vi "io_read_errors.vi"(8 "error in":errorcluster, 11 "VISA resource name":refnum<visa-resource-name>) -> (0 "error out":errorcluster, 3 "VISA resource name out":refnum<visa-resource-name>)   [LabVIEW 2014, in "rszvl_rsidr_core.lvlib"]
uses:
  rszvl_rsidr_core.lvlib
  type_Error_Codes.ctl
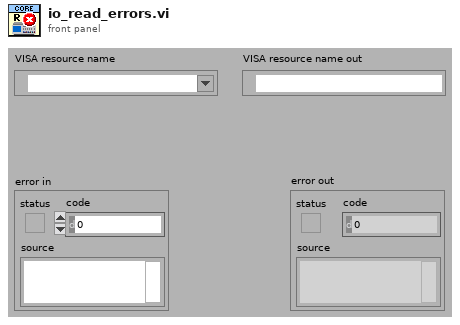
[diagram p1: front panel]
types:
  T1 = typedef "rszvl_rsidr_core.lvlib/type_Error_Codes.ctl" = enum16{"No_error", "VISA_err_ResourceNotFound", "VISA_err_Timeout", "VISA_warn_MoreDataAvailable", "RS_err_MissingCallback", "RS_err_InvalidAttribute", "RS_err_InvalidValue", "RS_err_UnknownResource", "RS_err_AlreadyInitialized", "RS_err_InstrumentStatus", "RS_err_BadRepCapName", "RS_err_TypesMismatch", "RS_err_ValueNotSupported", "RS_err_InvalidRngTable", "RS_err_IDqueryFail", "RS_err_UnexpResponse", "VISA_warn_ConfigNotLoaded", "RS_err_AttributeNotReadable", "RS_err_AttributeNotWritable", "RS_err_InstrumentType", "RS_err_InstrumentOption", "VISA_err_InvalidSize", "RS_err_ReliabilityIndicator", "VISA_warn_UnknownStatus", "VISA_warn_TermCharRead", "VISA_err_IO_error"}
  T2 = typedef "rszvl_rsidr_core.lvlib/type_Session_Data.ctl" = cluster{"Instr type":string, "Instr type for err. msg.":string, "Installed Options":string[], "OPC Timeout":i32, "Query Instrument Status":bool, "Check Range":bool, "Check Options":bool, "Add LF to Write":bool, "Simulate":bool, "Logging":bool, "Logging params":variant, "Interface Type":enum16{"Unknown", "GPIB", "VXI", "GPIB_VXI", "ASRL", "PXI", "TCPIP", "USB", "SOCKET"}, "Fast Sweep":i32, "AdditionalFlags":i32, "WaitBeforeWrite":i32, "WaitBeforeRead":i32, "BinDataChunkSize":i64}
  T3 = enum16{"Unknown", "GPIB", "VXI", "GPIB_VXI", "ASRL", "PXI", "TCPIP", "USB", "SOCKET"}
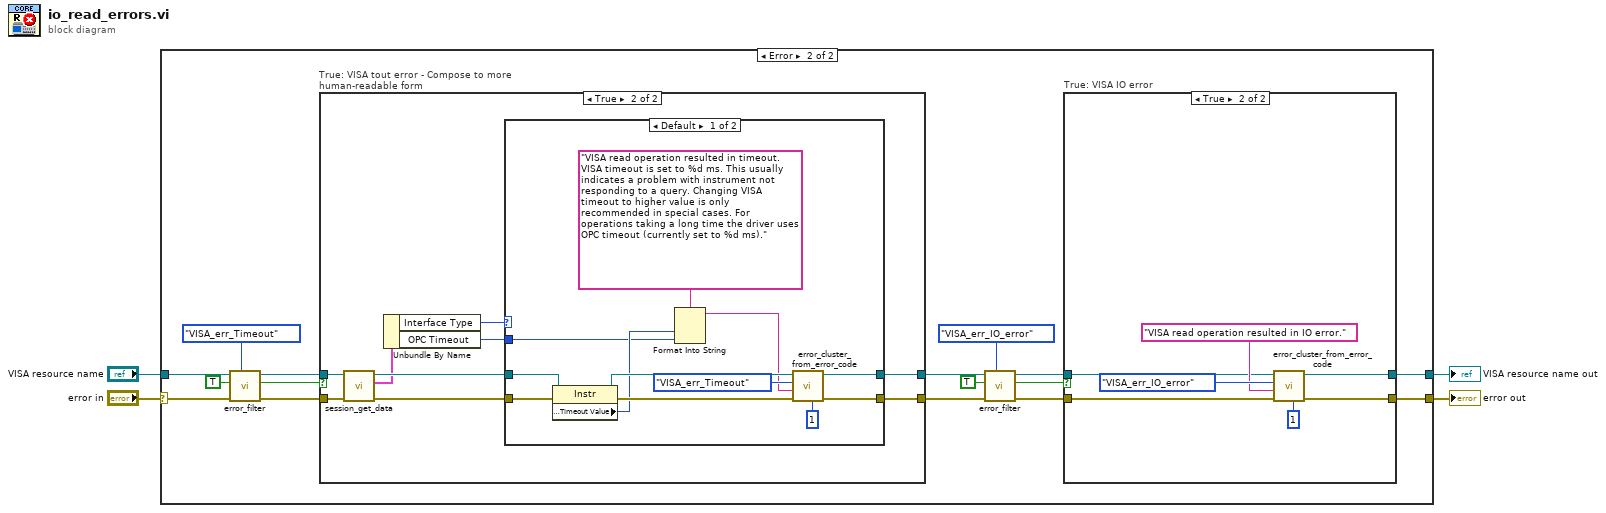
[diagram p0: block diagram]
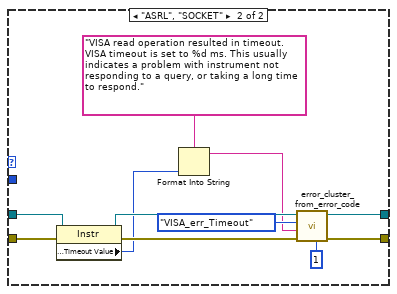
[diagram p5: hidden frame]
diagram:
  n1 = case shown="Error" "error in" {
    selector: "error in" -> [w6 w18]
    tunnel: [w6 w7] -> w2
    tunnel: "VISA resource name" -> [w5 w17]
    tunnel: [w5 w8] -> w1
    frame No Error {
    }
    frame Error {
      n2 = call "error_filter.vi"("Error Enum in"=type_Error_Codes."VISA_err_Timeout" ("Code to detect"), "error in"=w18, "Clear detected code (F)"=TRUE, "VISA resource name"=w17) -> ("error out"=w20:errorcluster, "Code Detected"=w19:bool, "VISA resource name out"=w16:refnum<visa-resource-name>)  [unwired: 5 in]
      n3 = case "True: VISA tout error - Compose to more human-readable form" shown="True" w19 {
        tunnel: w20 -> [w33 w40]
        tunnel: [w33 w42] -> w13
        tunnel: [w32 w41] -> w14
        tunnel: w16 -> [w32 w37]
        frame False {
        }
        frame True {
          n4 = call "session_get_data.vi"("error in"=w40, "VISA resource name"=w37) -> ("error out"=w39:errorcluster, "Session User Data out"=w36:T2, "VISA resource name out"=w38:refnum<visa-resource-name>)  [unwired: 7 in]
          n5 = Unbundle By Name(w36) -> ("Interface Type"=w34:T3, "OPC Timeout"=w35:i32)
          n6 = case shown="Default" w34 {
            tunnel: [w53 w64] -> w42
            tunnel: [w52 w63] -> w41
            tunnel: w39 -> [w46 w57]
            tunnel: w38 -> [w45 w56]
            tunnel: w35 -> [w44 _]
            frame Default {
              n7 = property on="Property Node" class="Instr"(reference=w45, error in=w46) -> (reference out=w50:refnum<visa-resource-name>, error out=w51:errorcluster, "General Settings:Timeout Value"=w49:u32)
              n8 = Format Into String(format string="VISA read operation resulted in timeout. VISA timeout is set to %d ms. This usually indicates a problem with instrument not responding to a query. Changing VISA timeout to higher value is only recommended in special cases. For operations taking a long time the driver uses OPC timeout (currently set to %d ms).", w49, w44) -> (resulting string=w48:string)  [unwired: 2 in, 1 out]
              n9 = call "error_cluster_from_error_code.vi"("Cut first x elements\nfrom Error Chain (0)"=1 ("Cut first x elements\nfrom Error Chain (0)"), "error in"=w51, "error message (\"\")"=w48, "Error Enum in"=type_Error_Codes."VISA_err_Timeout", "VISA resource name"=w50) -> ("error out"=w53:errorcluster, "VISA resource name out"=w52:refnum<visa-resource-name>)  [unwired: 5 in]
            }
            frame "ASRL", "SOCKET" {
              n10 = property on="Property Node" class="Instr"(reference=w56, error in=w57) -> (reference out=w61:refnum<visa-resource-name>, error out=w62:errorcluster, "General Settings:Timeout Value"=w60:u32)
              n11 = Format Into String(format string="VISA read operation resulted in timeout. VISA timeout is set to %d ms. This usually indicates a problem with instrument not responding to a query, or taking a long time to respond.", w60) -> (resulting string=w59:string)  [unwired: 2 in, 1 out]
              n12 = call "error_cluster_from_error_code.vi"("Cut first x elements\nfrom Error Chain (0)"=1 ("Cut first x elements\nfrom Error Chain (0)"), "error in"=w62, "error message (\"\")"=w59, "Error Enum in"=type_Error_Codes."VISA_err_Timeout", "VISA resource name"=w61) -> ("error out"=w64:errorcluster, "VISA resource name out"=w63:refnum<visa-resource-name>)  [unwired: 5 in]
            }
          }
        }
      }
      n13 = call "error_filter.vi"("Error Enum in"=type_Error_Codes."VISA_err_IO_error" ("Code to detect"), "error in"=w13, "Clear detected code (F)"=TRUE, "VISA resource name"=w14) -> ("error out"=w10:errorcluster, "Code Detected"=w9:bool, "VISA resource name out"=w11:refnum<visa-resource-name>)  [unwired: 5 in]
      n14 = case "True: VISA IO error" shown="True" w9 {
        tunnel: w10 -> [w23 w25]
        tunnel: [w24 w31] -> w8
        tunnel: w11 -> [w24 w26]
        tunnel: [w23 w30] -> w7
        frame False {
        }
        frame True {
          n15 = call "error_cluster_from_error_code.vi"("Cut first x elements\nfrom Error Chain (0)"=1 ("Cut first x elements\nfrom Error Chain (0)"), "error in"=w25, "error message (\"\")"="VISA read operation resulted in IO error.", "Error Enum in"=type_Error_Codes."VISA_err_IO_error", "VISA resource name"=w26) -> ("error out"=w30:errorcluster, "VISA resource name out"=w31:refnum<visa-resource-name>)  [unwired: 5 in]
        }
      }
    }
  }
  "VISA resource name out" <- w1
  "error out" <- w2
